vi "TSLIN_SetChannelCount.vi"(8 "错误输入（无错误）":errorcluster, 10 "Aount":i32, 11 "路径输入":path) -> (0 "错误输出":errorcluster, 3 "路径输出":path, 4 "Set_LIN_Channel_Count_Successfully":bool)   [LabVIEW 2019]
uses:
  Config/TSMaster.dll
panel:
  out "Set_LIN_Channel_Count_Successfully 2":bool
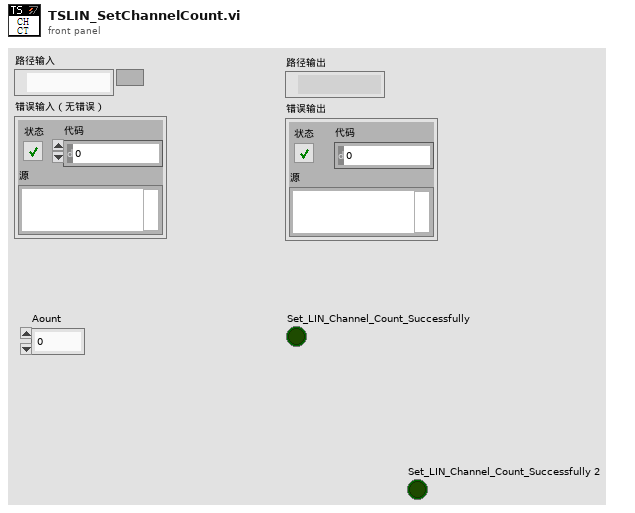
[diagram p1: front panel]
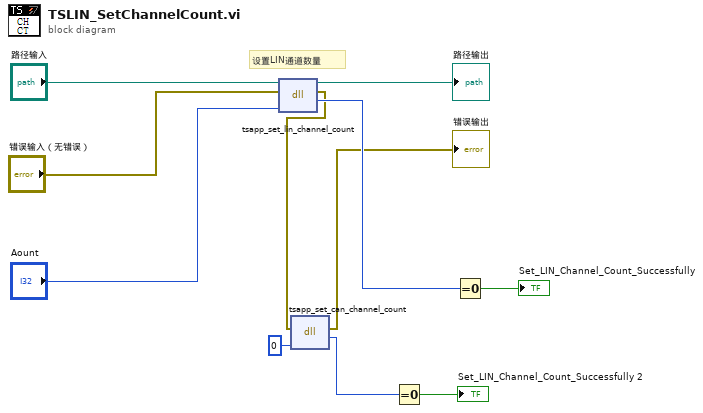
[diagram p0: block diagram]
diagram:
  # "设置LIN通道数量"
  n1 = dll-call lib="PTH2@abs EDemo同星TSCAN_V1.4_20220301ConfigTSMaster.dll" fn="tsapp_set_lin_channel_count"(path in="路径输入", error in="错误输入（无错误）", "Aount"="Aount") -> (path out=→"路径输出":path, error out=w5:errorcluster, "tsapp_set_can_channel_count"=w9:i32)  [unwired: 2 in]
  n2 = dll-call lib="C:/Users/XYY/Desktop/LabView Demo/TSCAN_LB2018_V1.4_20220309/Config/TSMaster.dll" fn="tsapp_set_can_channel_count"(error in=w5, "ACount"=0) -> (error out=→"错误输出":errorcluster, "返回类型"=w2:i32)  [unwired: 3 in, 1 out]
  n3 = Equal To 0?(x=w2) -> (x = 0?=→"Set_LIN_Channel_Count_Successfully 2":bool)
  n4 = Equal To 0?(x=w9) -> (x = 0?=→"Set_LIN_Channel_Count_Successfully":bool)
